vi "DSA Configuration.vi"(0 "Output Physical Channel":tag, 1 "Input  Physical Channel":tag, 5 "Sampling Rate [Hz]":dbl, 7 "interactive configuration dialog":bool, 9 "DSA channel settings":T1, 11 "error in":errorcluster) -> (4 "Output Task ID Out":refnum<k21>, 6 "Input Task ID Out":refnum<k21>, 10 "actual sample rate":dbl, 15 "error out":errorcluster)   [LabVIEW 2018]
uses:
  <vilib>/DAQmx/create/channels.llb/DAQmx Create Channel (AI-Voltage-Basic).vi
  <vilib>/DAQmx/configure/timing.llb/DAQmx Timing (Sample Clock).vi
  <vilib>/DAQmx/create/channels.llb/DAQmx Create Channel (AO-Voltage-Basic).vi
  <vilib>/DAQmx/configure/trigger.llb/DAQmx Start Trigger (Digital Edge).vi
  <resource>/objmgr/daqmx.rc
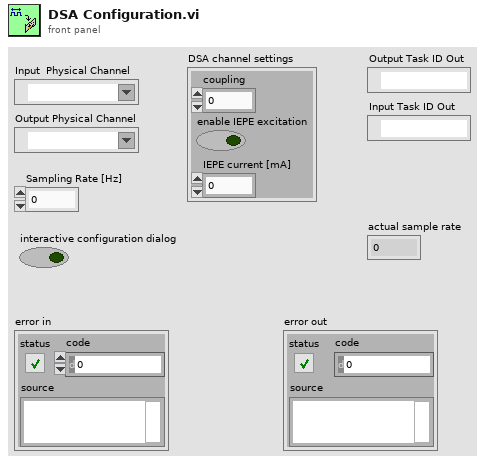
[diagram p1: front panel]
types:
  T1 = cluster{"coupling":i32, "enable IEPE excitation":bool, "IEPE current [mA]":dbl}
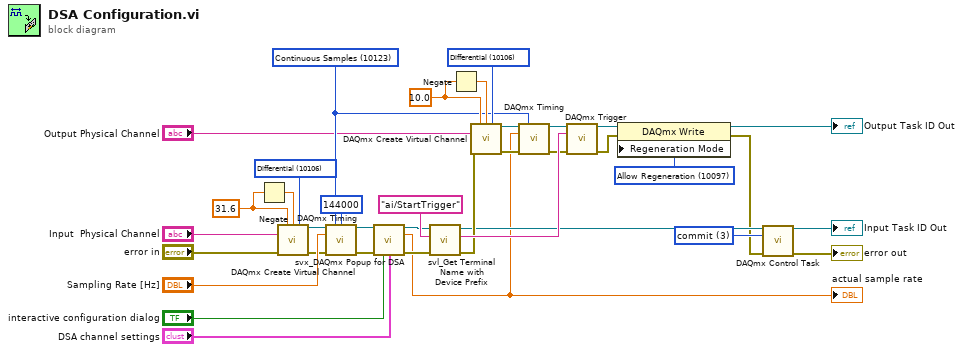
[diagram p0: block diagram]
diagram:
  w1 = 10106 items=["default"=-1, "RSE"=10083, "NRSE"=10078, "Differential"=10106, "Pseudodifferential"=12529] ("input terminal configuration")
  w11 = 3 items=["verify"=2, "reserve"=4, "commit"=3, "unreserve"=5, "abort"=6] ("action")
  w34 = 10.0 ("maximum value")
  w31 = 10106 items=["Default"=-1, "RSE"=10083, "Differential"=10106, "Pseudodifferential"=12529] ("output terminal configuration")
  w33 = 31.6 ("maximum value")
  w18 = 10097 items=["Allow Regeneration"=10097, "Do Not Allow Regeneration"=10158] ("RegenMode")
  w25 = 10123 items=["Finite Samples"=10178, "Continuous Samples"=10123] ("sample mode")
  n1 = Negate(x=w33) -> (-x=w32:dbl)
  n2 = call-poly <vilib>:"DAQmx Create Virtual Channel.vi"("maximum value"=w33, "minimum value"=w32, "input terminal configuration"=w1, "physical channels"="Input  Physical Channel", "error in"="error in") -> ("task out"=w19:refnum<k21>, "error out"=w20:errorcluster)  [unwired: 9 in]
  n3 = call-poly <vilib>:"DAQmx Timing.vi"("task/channels in"=w19, "sample mode"=w25, "samples per channel"=144000, "rate"="Sampling Rate [Hz]", "error in"=w20) -> ("task out"=w27:refnum<k21>, "error out"=w28:errorcluster)  [unwired: 9 in]
  n4 = call <vilib>:"svx_DAQmx Popup for DSA.vi"("task in"=w27, "error in (no error)"=w28, "interactive configuration dialog"="interactive configuration dialog", "DSA channel settings"="DSA channel settings") -> ("task out"=w22:refnum<k21>, "actual sample rate"=w5:dbl, "error out"=w23:errorcluster)  [unwired: 9 in]
  "actual sample rate" <- w5
  n5 = call <vilib>:"svl_Get Terminal Name with Device Prefix.vi"("error in (no error)"=w23, "local terminal name"="ai/StartTrigger", "task/channels in"=w22) -> ("error out"=w21:errorcluster, "terminal name with device prefix"=w26:tag, "task out"=w10:refnum<k21>)  [unwired: 6 in]
  n6 = Negate(x=w34) -> (-x=w35:dbl)
  n7 = call-poly <vilib>:"DAQmx Create Virtual Channel.vi"("maximum value"=w34, "minimum value"=w35, "output terminal configuration"=w31, "physical channels"="Output Physical Channel", "error in"=w21) -> ("task out"=w12:refnum<k21>, "error out"=w13:errorcluster)  [unwired: 9 in]
  n8 = call-poly <vilib>:"DAQmx Timing.vi"("task/channels in"=w12, "sample mode"=w25, "rate"=w5, "error in"=w13) -> ("task out"=w14:refnum<k21>, "error out"=w15:errorcluster)  [unwired: 10 in]
  n9 = call-poly <vilib>:"DAQmx Trigger.vi"("task/channels in"=w14, "source"=w26, "error in"=w15) -> ("task out"=w16:refnum<k21>, "error out"=w17:errorcluster)  [unwired: 11 in]
  n10 = property class="DAQmx Write"(reference=w16, error in=w17, "Regeneration Mode"=w18) -> (reference out=→"Output Task ID Out":refnum<k21>, error out=w9:errorcluster)
  n11 = call <vilib>:"DAQmx Control Task.vi"("task/channels in"=w10, "action"=w11, "error in"=w9) -> ("task out"=→"Input Task ID Out":refnum<k21>, "error out"=→"error out":errorcluster)  [unwired: 11 in]
